vi "SynchIO.TestLauncher.vi"() -> ()   [LabVIEW 2016, in "SynchIO.lvclass"]
doc: "JKI State Machine Objects (SMO) 1.0.0.5\nJKI - JKI\nCopyright (c) 2016, JKI"
uses:
  SynchIO.lvclass
  C:/Program Files (x86)/National Instruments/LabVIEW 2016/vi.lib/JKI/JKI SMO/SMO/SMO.lvclass
  <vilib>/JKI/JKI SMO/SMO/Typedefs/SMOState --Enum.ctl
  <vilib>/JKI/JKI SMO/SMO/SMO.lvclass
panel:
  out "Old Value":string
  out "New Value":string
  in  "Send":bool
  in  "Data":string
  out "error out":errorcluster
  in  "Stop":bool
  # "SMO Test Launcher"
  # "For instructions on how to use the JKI State Machine Objects, examples and video tutorials, visit:\nhttp://jki.net/state-machine-objects/\n\nJKI State Machine Objects™\nhttp://jki.net/state-machine-objects/\nCopyright (C) 2005-2015, JKI <info@jki.net>\nALL RIGHTS RESERVED"
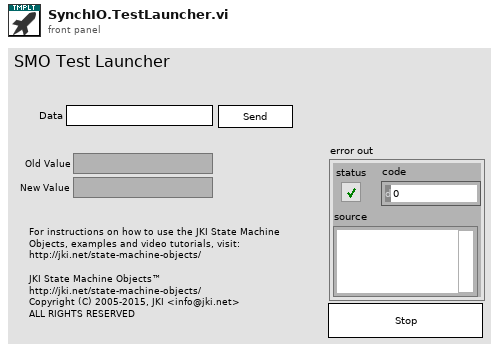
[diagram p1: front panel]
types:
  T1 = typedef "SynchIO.lvclass/PublicEvents--Cluster.ctl" = cluster{"Data Changed":refnum<user-event>}
  T2 = typedef "SMO.lvclass/Public Events.ctl" = cluster{"Error":refnum<user-event>, "State":refnum<user-event>}
  T3 = typedef "SMO.lvclass/SMOState --Enum.ctl" = enum16{"unknown", "Created", "Started", "Stopped"}
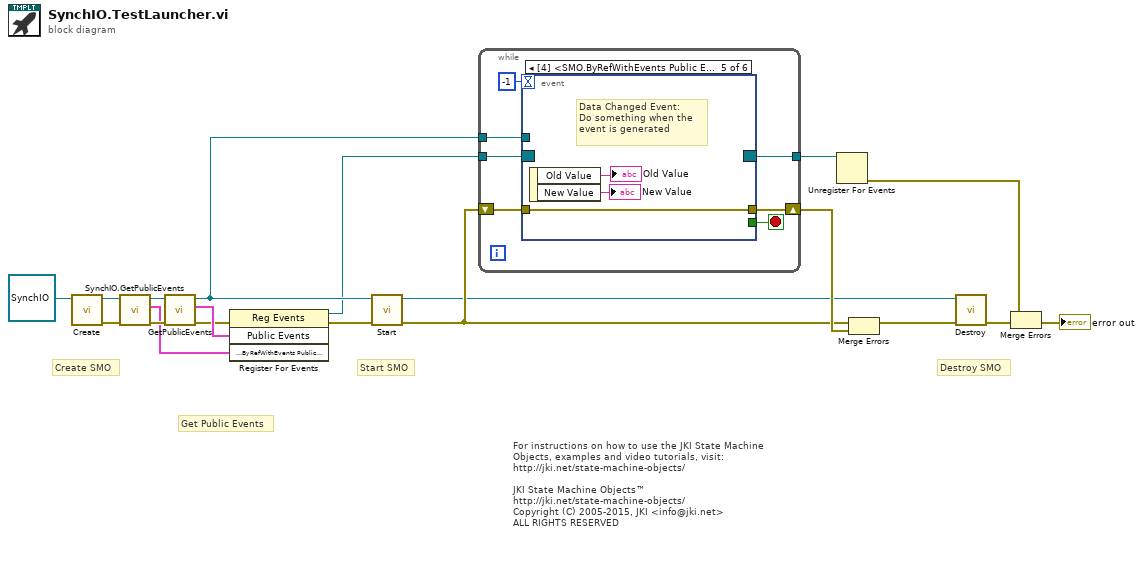
[diagram p0: block diagram]
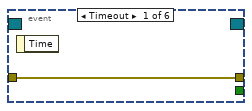
[diagram p2: hidden frame]
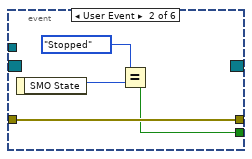
[diagram p3: hidden frame]
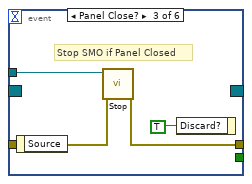
[diagram p4: hidden frame]
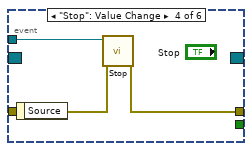
[diagram p5: hidden frame]
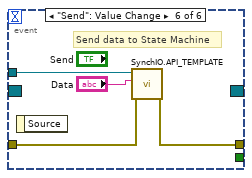
[diagram p6: hidden frame]
diagram:
  # "For instructions on how to use the JKI State Machine Objects, examples and video tutorials, visit:\nhttp://jki.net/state-machine-objects/\n\nJKI State Machine Objects™\nhttp://jki.net/state-machine-objects/\nCopyright (C) 2005-2015, JKI <info@jki.net>\nALL RIGHTS RESERVED"
  # "Get Public Events"
  # "Start SMO"
  # "Destroy SMO"
  # "Create SMO"
  n1 = call <vilib>:"Create.vi"("SMO"=refnum<class "SynchIO.lvclass"> refnum ("SMO.Template.lvclass")) -> ("error out"=w5:errorcluster, "SMO out"=w3:refnum<class "SynchIO.lvclass">)  [unwired: 8 in, 1 out]
  n2 = call "SynchIO.GetPublicEvents.vi"("error in (no error)"=w5, "SynchIO"=w3) -> ("error out"=w4:errorcluster, "SMO.ByRefWithEvents Public Events"=w1:T1, "SynchIO out"=w2:refnum<class "SynchIO.lvclass">)  [unwired: 7 in]
  n3 = call <vilib>:"GetPublicEvents.vi"("error in (no error)"=w4, "SMO"=w2) -> ("error out"=w7:errorcluster, "Public Events"=w8:T2, "SMO out"=w10:refnum<class "SynchIO.lvclass">)  [unwired: 7 in]
  n4 = register-events(error in=w7, w8, w1) -> (reference out=w6:refnum<event-registration>, error out=w9:errorcluster)  [unwired: 1 in]
  n5 = call <vilib>:"Start.vi"("error in (no error)"=w9, "SMO"=w10) -> ("error out"=w13:errorcluster, "SMO out"=w11:refnum<class "SynchIO.lvclass">)  [unwired: 8 in]
  n6 = while {
    shift-right: [w25] -> w18
    shift-left: w13 -> [w24]
    tunnel: w6 -> [w23]
    tunnel: [w22] -> w19
    tunnel: w10 -> [w21]
    stop <- w26 stop-if-true
    n7 = event shown="[4] <SMO.ByRefWithEvents Public Events.Data Changed>: User Event" {
      selector: w23 -> [_ _ _ _ _ _]
      dyn-events: [_ _ _ _ _ _] -> w22
      timeout: -1 -> [_ _ _ _ _ _]
      tunnel: [_ w28 _ _ _ _] -> w26
      tunnel: w21 -> [_ _ w35 w38 _ w45]
      tunnel: [w27 w31 w34 w37 w41 w42] -> w25
      tunnel: w24 -> [w27 w31 w33 w36 w41 w43]
      event Timeout {
        n8 = event-data() -> ()  [unwired: 1 in, 1 out]
      }
      event User Event {
        n9 = event-data() -> ("SMO State"=w30:T3)  [unwired: 1 in]
        n10 = Equal?(x=SMOState_--Enum."Stopped", y=w30) -> (x = y?=w28:bool)
      }
      event Panel Close? {
        # "Stop SMO if Panel Closed"
        n11 = event-data() -> ()  [unwired: 1 in, 1 out]
        n12 = call <vilib>:"Stop.vi"("error in (no error)"=w33, "SMO"=w35) -> ("error out"=w34:errorcluster)  [unwired: 8 in, 1 out]
        n13 = event-data("Discard?"=TRUE ("OK")) -> ()  [unwired: 1 in, 1 out]
      }
      event "Stop": Value Change {
        n14 = event-data() -> ()  [unwired: 1 in, 1 out]
        n15 = call <vilib>:"Stop.vi"("error in (no error)"=w36, "SMO"=w38) -> ("error out"=w37:errorcluster)  [unwired: 8 in, 1 out]
      }
      event User Event {
        # "Data Changed Event:\nDo something when the\nevent is generated"
        n16 = event-data() -> ("Old Value"=→"Old Value":string, "New Value"=→"New Value":string)  [unwired: 1 in]
      }
      event "Send": Value Change {
        # "Send data to State Machine"
        n17 = event-data() -> ()  [unwired: 1 in, 1 out]
        n18 = call "SynchIO.API_TEMPLATE.vi"("error in (no error)"=w43, "myData"="Data", "SynchIO"=w45) -> ("error out"=w42:errorcluster)  [unwired: 6 in, 2 out]
      }
    }
  }
  n19 = Unregister For Events(event registration refnum=w19) -> (error out=w17:errorcluster)  [unwired: 1 in]
  n20 = Merge Errors(w13, w18) -> (w12:errorcluster)
  n21 = call <vilib>:"Destroy.vi"("error in (no error)"=w12, "SMO"=w11) -> ("error out"=w15:errorcluster)  [unwired: 9 in]
  n22 = Merge Errors(w17, w15) -> (→"error out":errorcluster)
